vi "Prepare_Query_String.vi"(1 "Input String":string) -> (0 "Output String":string)   [LabVIEW 2011]
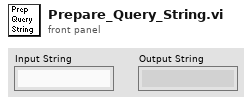
[diagram p1: front panel]
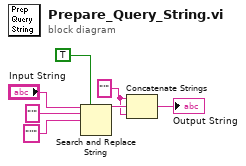
[diagram p0: block diagram]
diagram:
  w2 = "'" ("string")
  n1 = Search and Replace String(replace all?=TRUE ("replace all? (F)"), input string="Input String", search string="'", replace string="''" ("replace string (\"\")")) -> (result string=w3:string)  [unwired: 4 in, 3 out]
  n2 = Concatenate Strings(w2, w3, w2) -> (→"Output String":string)
